vi "Goo0FF.vi"(10 "ColorSensor":dbl[](array[numeric])=[2.7490231560000002, 2.873534862, 2.8564450200000002, 2.873534862], 11 "클러스터":T1={{"정지할 차이값"=0.08, "흰색과 밖 차이값"=0.15, "흰/검 반 값 "=0.3}, {"4: 오른각도"=122.0, "4: 뒷쪽각도"=0.0, "5: 오른각도"=120.0, "5: 앞쪽각도"=245.0, "6: 왼쪽각도"=245.0, "6: 앞쪽각도"=120.0}, {"2: 공각도"=233.0, "2: 굴릴각도"=60.0}}) -> ()   [LabVIEW 2014]
uses:
  <vilib>/myRIO/Instrument Drivers/Onboard IO/AI/vis/Read.vi
  <vilib>/myRIO/Instrument Drivers/Onboard IO/AI/vis/Smart Open.vi
  <vilib>/Utility/error.llb/Error Cluster From Error Code.vi
  <vilib>/myRIO/Common/Instrument Driver Framework/myRIO v1.0/AI/vis/myRIO v1.0 Read AI.vi
panel:
  in  "오른쪽맞추는 초":u32=7000
  in  "오른쪽으로":u32=1000
  in  "왼쪽차이":dbl=0.25
  in  "Servo Position2 (0 - 255)":u8(slide)=115 step=1 scale=0.0..255.0
  in  "왼쪽가는 시간":u32=250
  in  "뒤로가는 시간":u32=100
  in  "Select Servo 2":string(combo)="Servo 2"
  in  "1: 정지":u8=128
  in  "1: 내리기":u8=10
  in  "1: 내리는 시간":u32=4000
  in  "Select Servo":string(combo)="Servo 1"
  in  "Select Servo 6":string(combo)="Servo 6"
  in  "Select Servo 5":string(combo)="Servo 5"
  in  "Select Servo 4":string(combo)="Servo 4"
  in  "서브 컨트롤":u8=1
  out "흰색과 밖 차이값":dbl=0.15
  # "마지막! 되돌아가기"
  # "115\n2번서브모터 본래방향"
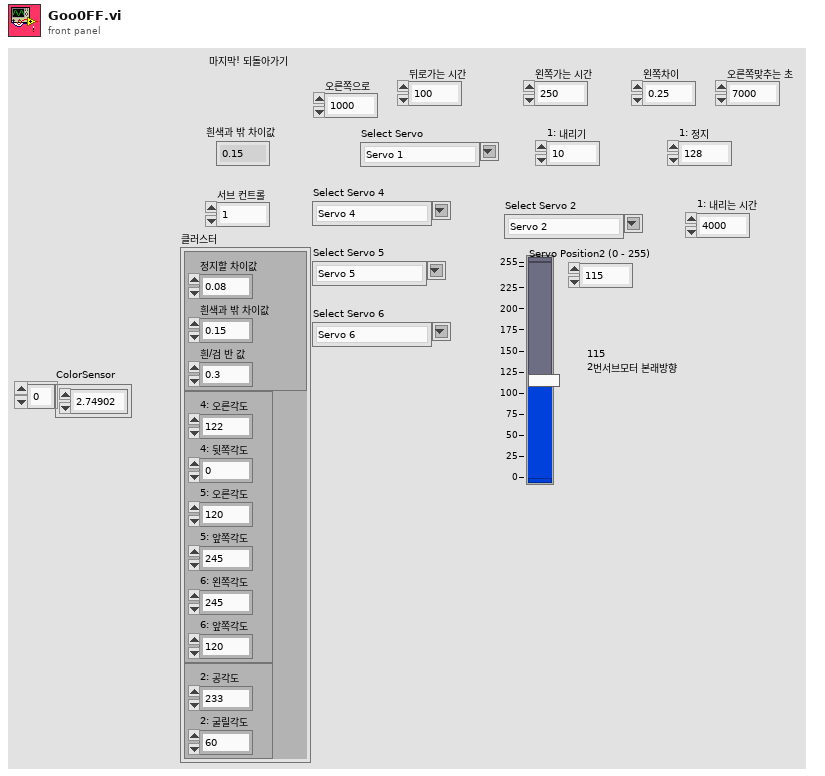
[diagram p1: front panel]
types:
  T1 = cluster{cluster{"정지할 차이값":dbl, "흰색과 밖 차이값":dbl, "흰/검 반 값 ":dbl}, cluster{"4: 오른각도":dbl, "4: 뒷쪽각도":dbl, "5: 오른각도":dbl, "5: 앞쪽각도":dbl, "6: 왼쪽각도":dbl, "6: 앞쪽각도":dbl}, cluster{"2: 공각도":dbl, "2: 굴릴각도":dbl}}
  T2 = cluster{"4: 오른각도":dbl, "4: 뒷쪽각도":dbl, "5: 오른각도":dbl, "5: 앞쪽각도":dbl, "6: 왼쪽각도":dbl, "6: 앞쪽각도":dbl}
  T3 = cluster{"정지할 차이값":dbl, "흰색과 밖 차이값":dbl, "흰/검 반 값 ":dbl}
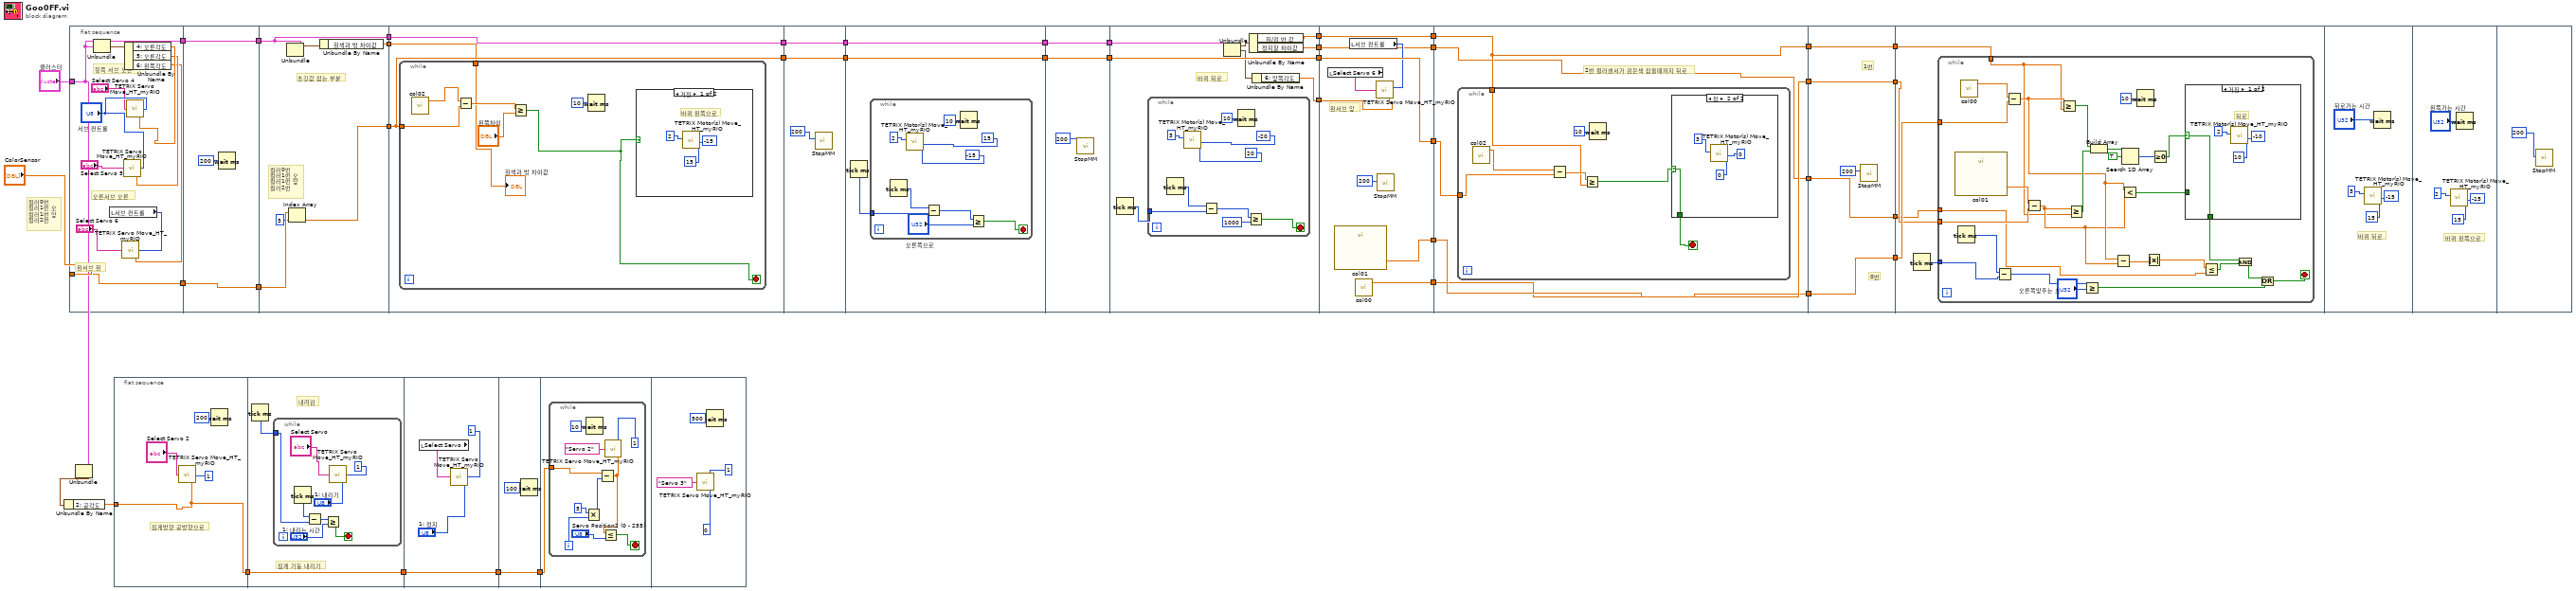
[diagram p0: block diagram]
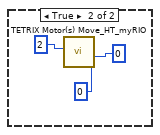
[diagram p2: hidden frame]
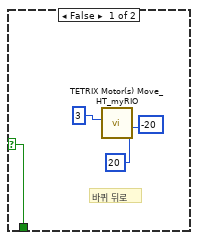
[diagram p3: hidden frame]
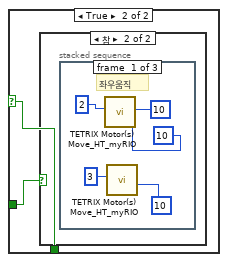
[diagram p4: hidden frame]
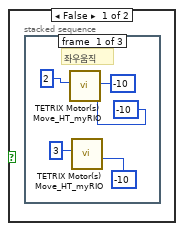
[diagram p5: hidden frame]
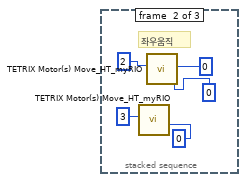
[diagram p6: hidden frame]
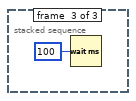
[diagram p7: hidden frame]
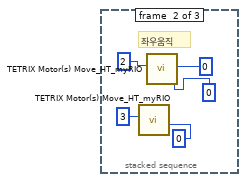
[diagram p8: hidden frame]
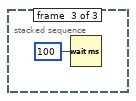
[diagram p9: hidden frame]
diagram:
  # "컬러0번\n컬러1번 오\n컬러1번 앞\n컬러2번"
  n1 = flat-sequence {
    tunnel: [w41] -> _
    tunnel: "클러스터" -> [w41]
    tunnel: [w42] -> w26
    tunnel: "ColorSensor" -> [w42]
    tunnel: [w41] -> w23
    tunnel: [w53] -> w27
    tunnel: w26 -> [w53]
    tunnel: [w52] -> w24
    tunnel: w23 -> [w52]
    tunnel: [w58] -> w40
    tunnel: w27 -> [w60]
    tunnel: w24 -> [w55]
    tunnel: [w56] -> w22
    tunnel: [w55] -> w21
    tunnel: w40 -> [w63]
    tunnel: [w63] -> w37
    tunnel: w22 -> [w62]
    tunnel: w21 -> [w61]
    tunnel: [w61] -> w20
    tunnel: w37 -> [w79]
    tunnel: [w79] -> w35
    tunnel: w20 -> [w77]
    tunnel: [w77] -> w19
    tunnel: w35 -> [w82]
    tunnel: [w82] -> w34
    tunnel: w19 -> [w81]
    tunnel: [w81] -> w18
    tunnel: w34 -> [w94]
    tunnel: [w94] -> w33
    tunnel: w18 -> [w92]
    tunnel: [w92] -> w17
    tunnel: w33 -> [w101]
    tunnel: [w101] -> w38
    tunnel: w17 -> [w100]
    tunnel: [w99] -> w16
    tunnel: [w96] -> w14
    tunnel: [w95] -> w3
    tunnel: [w120] -> w39
    tunnel: w38 -> [w120]
    tunnel: [w119] -> w36
    tunnel: [w118] -> w32
    tunnel: w16 -> [w114]
    tunnel: [w113] -> w15
    tunnel: w14 -> [w113]
    tunnel: [w112] -> w4
    tunnel: w3 -> [w112]
    tunnel: w39 -> [w125]
    tunnel: w36 -> [w124]
    tunnel: w32 -> [w123]
    tunnel: [w124] -> w30
    tunnel: [w123] -> w28
    tunnel: w15 -> [w122]
    tunnel: [w122] -> w5
    tunnel: w4 -> [w121]
    tunnel: [w121] -> w2
    tunnel: [w145] -> w31
    tunnel: w30 -> [w145]
    tunnel: [w144] -> w29
    tunnel: w28 -> [w144]
    tunnel: [w142] -> w6
    tunnel: w5 -> [w142]
    tunnel: w2 -> [w141]
    tunnel: [w141] -> w1
    tunnel: w31 -> [w149]
    tunnel: w29 -> [w150]
    tunnel: w6 -> [w148]
    tunnel: w1 -> [w147]
    frame #0 {
      # "왼서브 왼"
      # "오른서브 오른"
      # "뒷쪽 서브 오른"
      n2 = Unbundle(w41) -> (w46:T2)  [unwired: 2 out]
      n3 = local read "서브 컨트롤"() -> (w51:u8)
      n4 = Unbundle By Name(w46) -> ("4: 오른각도"=w45:dbl, "5: 오른각도"=w44:dbl, "6: 왼쪽각도"=w43:dbl)
      n5 = call <vilib>:"TETRIX Servo Move_HT_myRIO.vi"("Servo Position (0 - 255)"=w43, "Controller Daisy Chain Position (1 - 4)"=w51, "Select Servo"="Select Servo 6") -> ()  [unwired: 2 in, 1 out]
      n6 = call <vilib>:"TETRIX Servo Move_HT_myRIO.vi"("Servo Position (0 - 255)"=w44, "Controller Daisy Chain Position (1 - 4)"="서브 컨트롤", "Select Servo"="Select Servo 5") -> ()  [unwired: 2 in, 1 out]
      n7 = call <vilib>:"TETRIX Servo Move_HT_myRIO.vi"("Servo Position (0 - 255)"=w45, "Controller Daisy Chain Position (1 - 4)"="서브 컨트롤", "Select Servo"="Select Servo 4") -> ()  [unwired: 2 in, 1 out]
    }
    frame #1 {
      n8 = Wait (ms)(milliseconds to wait=u32 200 ("대기 시간(ms)")) -> ()  [unwired: 1 out]
    }
    frame #2 {
      # "컬러0번\n컬러1번 오\n컬러1번 앞\n컬러2번"
      # "초깃값 잡는 부분"
      n9 = Unbundle(w55) -> (w57:T3)  [unwired: 2 out]
      n10 = Index Array(array=w60, index=3 ("인덱스")) -> (element=w58:dbl)
      n11 = Unbundle By Name(w57) -> ("흰색과 밖 차이값"=w56:dbl)
    }
    frame #3 {
      n12 = while {
        tunnel: w63 -> [w70]
        tunnel: w62 -> [w64]
        stop <- w66 stop-if-true
        n13 = call "col02.vi"() -> ("Col02 (B/AI2 (Pin 7))"=w67:dbl)  [unwired: 26 in, 1 out]
        n14 = Subtract(x=w67, y=w70) -> (x-y=w69:dbl)
        n15 = Greater Or Equal?(x=w69, y="왼쪽차이") -> (x >= y?=w66:bool)
        n16 = Wait (ms)(milliseconds to wait=u32 10 ("대기 시간(ms)")) -> ()  [unwired: 1 out]
        n17 = case shown="거짓" w66 {
          frame False {
            # "바퀴 왼쪽으로"
            n18 = call <vilib>:"TETRIX Motor(s) Move_HT_myRIO.vi"("Motor 2 Power (-100 to 100)\n0 = Stop/Brake\n-128 = Stop/Coast"=i8 15 ("Motor 2 Power (-100 to 100)\n0 = Stop/Brake\n-128 = Stop/Coast"), "Motor 1 Power (-100 to 100)\n0 = Stop/Brake\n-128 = Stop/Coast"=i8 -15 ("Motor 1 Power (-100 to 100)\n0 = Stop/Brake\n-128 = Stop/Coast"), "Controller Daisy Chain Position: 1 - 4"=u8 2) -> ()  [unwired: 6 in, 1 out]
          }
          frame True {
            n19 = call <vilib>:"TETRIX Motor(s) Move_HT_myRIO.vi"("Motor 2 Power (-100 to 100)\n0 = Stop/Brake\n-128 = Stop/Coast"=i8 0 ("Motor 2 Power (-100 to 100)\n0 = Stop/Brake\n-128 = Stop/Coast"), "Motor 1 Power (-100 to 100)\n0 = Stop/Brake\n-128 = Stop/Coast"=i8 0 ("Motor 1 Power (-100 to 100)\n0 = Stop/Brake\n-128 = Stop/Coast"), "Controller Daisy Chain Position: 1 - 4"=u8 2) -> ()  [unwired: 6 in, 1 out]
          }
        }
        "흰색과 밖 차이값" <- w64
      }
    }
    frame #4 {
      n20 = call "StopMM.vi"("대기 시간(ms)"=u32 200) -> ()  [unwired: 11 in]
    }
    frame #5 {
      n21 = Tick Count (ms)() -> (millisecond timer value=w80:u32)
      n22 = while {
        tunnel: w80 -> [w87]
        stop <- w85 stop-if-true
        n23 = Tick Count (ms)() -> (millisecond timer value=w88:u32)
        n24 = call <vilib>:"TETRIX Motor(s) Move_HT_myRIO.vi"("Motor 2 Power (-100 to 100)\n0 = Stop/Brake\n-128 = Stop/Coast"=i8 -15 ("Motor 2 Power (-100 to 100)\n0 = Stop/Brake\n-128 = Stop/Coast"), "Motor 1 Power (-100 to 100)\n0 = Stop/Brake\n-128 = Stop/Coast"=i8 15 ("Motor 1 Power (-100 to 100)\n0 = Stop/Brake\n-128 = Stop/Coast"), "Controller Daisy Chain Position: 1 - 4"=u8 2) -> ()  [unwired: 6 in, 1 out]
        n25 = Subtract(x=w88, y=w87) -> (x-y=w86:u32)
        n26 = Wait (ms)(milliseconds to wait=u32 10 ("대기 시간(ms)")) -> ()  [unwired: 1 out]
        n27 = Greater Or Equal?(x=w86, y="오른쪽으로") -> (x >= y?=w85:bool)
      }
    }
    frame #6 {
      n28 = call "StopMM.vi"("대기 시간(ms)"=u32 200) -> ()  [unwired: 11 in]
    }
    frame #7 {
      # "바퀴 뒤로"
      n29 = Tick Count (ms)() -> (millisecond timer value=w102:u32)
      n30 = while {
        tunnel: w102 -> [w107]
        stop <- w104 stop-if-true
        n31 = Tick Count (ms)() -> (millisecond timer value=w108:u32)
        n32 = call <vilib>:"TETRIX Motor(s) Move_HT_myRIO.vi"("Motor 2 Power (-100 to 100)\n0 = Stop/Brake\n-128 = Stop/Coast"=i8 20 ("Motor 2 Power (-100 to 100)\n0 = Stop/Brake\n-128 = Stop/Coast"), "Motor 1 Power (-100 to 100)\n0 = Stop/Brake\n-128 = Stop/Coast"=i8 -20 ("Motor 1 Power (-100 to 100)\n0 = Stop/Brake\n-128 = Stop/Coast"), "Controller Daisy Chain Position: 1 - 4"=u8 3) -> ()  [unwired: 6 in, 1 out]
        n33 = Subtract(x=w108, y=w107) -> (x-y=w106:u32)
        n34 = Wait (ms)(milliseconds to wait=u32 10 ("대기 시간(ms)")) -> ()  [unwired: 1 out]
        n35 = Greater Or Equal?(x=w106, y=u32 1000) -> (x >= y?=w104:bool)
      }
      n36 = Unbundle(w100) -> (w97:T3, w98:T2)  [unwired: 1 out]
      n37 = Unbundle By Name(w97) -> ("흰/검 반 값"=w96:dbl, "정지할 차이값"=w95:dbl)
      n38 = Unbundle By Name(w98) -> ("6: 앞쪽각도"=w99:dbl)
    }
    frame #8 {
      # "왼서브 앞"
      n39 = local read "Select Servo 6"() -> (w116:string)
      n40 = call "col01.vi"() -> ("Col01 (B/AI1 (Pin 5))"=w119:dbl)  [unwired: 26 in, 1 out]
      n41 = local read "서브 컨트롤"() -> (w117:u8)
      n42 = call "col00.vi"() -> ("Col00 (B/AI0 (Pin 3))"=w118:dbl)  [unwired: 26 in, 1 out]
      n43 = call <vilib>:"TETRIX Servo Move_HT_myRIO.vi"("Servo Position (0 - 255)"=w114, "Controller Daisy Chain Position (1 - 4)"=w117, "Select Servo"=w116) -> ()  [unwired: 2 in, 1 out]
      n44 = call "StopMM.vi"("대기 시간(ms)"=u32 200) -> ()  [unwired: 11 in]
    }
    frame #9 {
      # "2번 컬러센서가 검은색 잡을때까지 뒤로"
      n45 = while {
        tunnel: w125 -> [w131]
        tunnel: w122 -> [w127]
        stop <- w126 stop-if-true
        n46 = call "col02.vi"() -> ("Col02 (B/AI2 (Pin 7))"=w130:dbl)  [unwired: 26 in, 1 out]
        n47 = Subtract(x=w130, y=w131) -> (x-y=w129:dbl)
        n48 = Greater Or Equal?(x=w129, y=w127) -> (x >= y?=w128:bool)
        n49 = Wait (ms)(milliseconds to wait=u32 10 ("대기 시간(ms)")) -> ()  [unwired: 1 out]
        n50 = case shown="참" w128 {
          selector: w128 -> [w133 w137]
          tunnel: [w133 w137] -> w126
          frame False {
            # "바퀴 뒤로"
            n51 = call <vilib>:"TETRIX Motor(s) Move_HT_myRIO.vi"("Motor 2 Power (-100 to 100)\n0 = Stop/Brake\n-128 = Stop/Coast"=i8 20 ("Motor 2 Power (-100 to 100)\n0 = Stop/Brake\n-128 = Stop/Coast"), "Motor 1 Power (-100 to 100)\n0 = Stop/Brake\n-128 = Stop/Coast"=i8 -20 ("Motor 1 Power (-100 to 100)\n0 = Stop/Brake\n-128 = Stop/Coast"), "Controller Daisy Chain Position: 1 - 4"=u8 3) -> ()  [unwired: 6 in, 1 out]
          }
          frame True {
            n52 = call <vilib>:"TETRIX Motor(s) Move_HT_myRIO.vi"("Motor 2 Power (-100 to 100)\n0 = Stop/Brake\n-128 = Stop/Coast"=i8 0 ("Motor 2 Power (-100 to 100)\n0 = Stop/Brake\n-128 = Stop/Coast"), "Motor 1 Power (-100 to 100)\n0 = Stop/Brake\n-128 = Stop/Coast"=i8 0 ("Motor 1 Power (-100 to 100)\n0 = Stop/Brake\n-128 = Stop/Coast"), "Controller Daisy Chain Position: 1 - 4"=u8 3) -> ()  [unwired: 6 in, 1 out]
          }
        }
      }
    }
    frame #10 {
      # "0번"
      # "1번"
      n53 = call "StopMM.vi"("대기 시간(ms)"=u32 200) -> ()  [unwired: 11 in]
    }
    frame #11 {
      n54 = Tick Count (ms)() -> (millisecond timer value=w146:u32)
      n55 = while {
        tunnel: w149 -> [w176]
        tunnel: w150 -> [w174]
        tunnel: w148 -> [w160]
        tunnel: w147 -> [w159]
        tunnel: w146 -> [w156]
        stop <- w153 stop-if-true
        n56 = call "col01.vi"() -> ("Col01 (B/AI1 (Pin 5))"=w177:dbl)  [unwired: 26 in, 1 out]
        n57 = Tick Count (ms)() -> (millisecond timer value=w157:u32)
        n58 = call "col00.vi"() -> ("Col00 (B/AI0 (Pin 3))"=w175:dbl)  [unwired: 26 in, 1 out]
        n59 = Subtract(x=w157, y=w156) -> (x-y=w155:u32)
        n60 = Subtract(x=w175, y=w174) -> (x-y=w163:dbl)
        n61 = Subtract(x=w177, y=w176) -> (x-y=w162:dbl)
        n62 = Greater Or Equal?(x=w163, y=w160) -> (x >= y?=w173:bool)
        n63 = Greater Or Equal?(x=w162, y=w160) -> (x >= y?=w172:bool)
        n64 = Greater Or Equal?(x=w155, y="오른쪽맞추는 초") -> (x >= y?=w152:bool)
        n65 = Build Array(w173, w172) -> (w171:bool[])
        n66 = Subtract(x=w163, y=w162) -> (x-y=w166:dbl)
        n67 = Search 1D Array(1D array=w171, element=TRUE ("원소")) -> (index of element=w169:i32)  [unwired: 1 in]
        n68 = Less?(x=w163, y=w162) -> (x < y?=w161:bool)
        n69 = Wait (ms)(milliseconds to wait=u32 10 ("대기 시간(ms)")) -> ()  [unwired: 1 out]
        n70 = Absolute Value(x=w166) -> (abs(x)=w165:dbl)
        n71 = Greater Or Equal To 0?(x=w169) -> (x >= 0?=w164:bool)
        n72 = case shown="거짓" w164 {
          selector: w164 -> [w178 w182]
          tunnel: w161 -> [_ w183]
          tunnel: [w178 w182] -> w158
          frame False {
            # "뒤로"
            n73 = call <vilib>:"TETRIX Motor(s) Move_HT_myRIO.vi"("Motor 2 Power (-100 to 100)\n0 = Stop/Brake\n-128 = Stop/Coast"=i8 10 ("Motor 2 Power (-100 to 100)\n0 = Stop/Brake\n-128 = Stop/Coast"), "Motor 1 Power (-100 to 100)\n0 = Stop/Brake\n-128 = Stop/Coast"=i8 -10 ("Motor 1 Power (-100 to 100)\n0 = Stop/Brake\n-128 = Stop/Coast"), "Controller Daisy Chain Position: 1 - 4"=u8 2) -> ()  [unwired: 6 in, 1 out]
          }
          frame True {
            n74 = case shown="참" w183 {
              frame False {
                n75 = stacked-sequence {
                  frame #0 {
                    # "좌우움직"
                    n76 = call <vilib>:"TETRIX Motor(s) Move_HT_myRIO.vi"("Motor 2 Power (-100 to 100)\n0 = Stop/Brake\n-128 = Stop/Coast"=i8 -10 ("Motor 2 Power (-100 to 100)\n0 = Stop/Brake\n-128 = Stop/Coast"), "Motor 1 Power (-100 to 100)\n0 = Stop/Brake\n-128 = Stop/Coast"=i8 -10 ("Motor 1 Power (-100 to 100)\n0 = Stop/Brake\n-128 = Stop/Coast"), "Controller Daisy Chain Position: 1 - 4"=u8 2) -> ()  [unwired: 6 in, 1 out]
                    n77 = call <vilib>:"TETRIX Motor(s) Move_HT_myRIO.vi"("Motor 1 Power (-100 to 100)\n0 = Stop/Brake\n-128 = Stop/Coast"=i8 -10 ("Motor 1 Power (-100 to 100)\n0 = Stop/Brake\n-128 = Stop/Coast"), "Controller Daisy Chain Position: 1 - 4"=u8 3) -> ()  [unwired: 7 in, 1 out]
                  }
                  frame #1 {
                    # "좌우움직"
                    n78 = call <vilib>:"TETRIX Motor(s) Move_HT_myRIO.vi"("Motor 1 Power (-100 to 100)\n0 = Stop/Brake\n-128 = Stop/Coast"=i8 0 ("Motor 1 Power (-100 to 100)\n0 = Stop/Brake\n-128 = Stop/Coast"), "Controller Daisy Chain Position: 1 - 4"=u8 3) -> ()  [unwired: 7 in, 1 out]
                    n79 = call <vilib>:"TETRIX Motor(s) Move_HT_myRIO.vi"("Motor 2 Power (-100 to 100)\n0 = Stop/Brake\n-128 = Stop/Coast"=i8 0 ("Motor 2 Power (-100 to 100)\n0 = Stop/Brake\n-128 = Stop/Coast"), "Motor 1 Power (-100 to 100)\n0 = Stop/Brake\n-128 = Stop/Coast"=i8 0 ("Motor 1 Power (-100 to 100)\n0 = Stop/Brake\n-128 = Stop/Coast"), "Controller Daisy Chain Position: 1 - 4"=u8 2) -> ()  [unwired: 6 in, 1 out]
                  }
                  frame #2 {
                    n80 = Wait (ms)(milliseconds to wait=u32 100 ("대기 시간(ms)")) -> ()  [unwired: 1 out]
                  }
                }
              }
              frame True {
                n81 = stacked-sequence {
                  frame #0 {
                    # "좌우움직"
                    n82 = call <vilib>:"TETRIX Motor(s) Move_HT_myRIO.vi"("Motor 2 Power (-100 to 100)\n0 = Stop/Brake\n-128 = Stop/Coast"=i8 10 ("Motor 2 Power (-100 to 100)\n0 = Stop/Brake\n-128 = Stop/Coast"), "Motor 1 Power (-100 to 100)\n0 = Stop/Brake\n-128 = Stop/Coast"=i8 10 ("Motor 1 Power (-100 to 100)\n0 = Stop/Brake\n-128 = Stop/Coast"), "Controller Daisy Chain Position: 1 - 4"=u8 2) -> ()  [unwired: 6 in, 1 out]
                    n83 = call <vilib>:"TETRIX Motor(s) Move_HT_myRIO.vi"("Motor 1 Power (-100 to 100)\n0 = Stop/Brake\n-128 = Stop/Coast"=i8 10 ("Motor 1 Power (-100 to 100)\n0 = Stop/Brake\n-128 = Stop/Coast"), "Controller Daisy Chain Position: 1 - 4"=u8 3) -> ()  [unwired: 7 in, 1 out]
                  }
                  frame #1 {
                    # "좌우움직"
                    n84 = call <vilib>:"TETRIX Motor(s) Move_HT_myRIO.vi"("Motor 1 Power (-100 to 100)\n0 = Stop/Brake\n-128 = Stop/Coast"=i8 0 ("Motor 1 Power (-100 to 100)\n0 = Stop/Brake\n-128 = Stop/Coast"), "Controller Daisy Chain Position: 1 - 4"=u8 3) -> ()  [unwired: 7 in, 1 out]
                    n85 = call <vilib>:"TETRIX Motor(s) Move_HT_myRIO.vi"("Motor 2 Power (-100 to 100)\n0 = Stop/Brake\n-128 = Stop/Coast"=i8 0 ("Motor 2 Power (-100 to 100)\n0 = Stop/Brake\n-128 = Stop/Coast"), "Motor 1 Power (-100 to 100)\n0 = Stop/Brake\n-128 = Stop/Coast"=i8 0 ("Motor 1 Power (-100 to 100)\n0 = Stop/Brake\n-128 = Stop/Coast"), "Controller Daisy Chain Position: 1 - 4"=u8 2) -> ()  [unwired: 6 in, 1 out]
                  }
                  frame #2 {
                    n86 = Wait (ms)(milliseconds to wait=u32 100 ("대기 시간(ms)")) -> ()  [unwired: 1 out]
                  }
                }
              }
            }
          }
        }
        n87 = Less Or Equal?(x=w165, y=w159) -> (x <= y?=w167:bool)
        n88 = And(x=w158, y=w167) -> (x .and. y?=w154:bool)
        n89 = Or(x=w154, y=w152) -> (x .or. y?=w153:bool)
      }
    }
    frame #12 {
      # "바퀴 뒤로"
      n90 = call <vilib>:"TETRIX Motor(s) Move_HT_myRIO.vi"("Motor 2 Power (-100 to 100)\n0 = Stop/Brake\n-128 = Stop/Coast"=i8 15 ("Motor 2 Power (-100 to 100)\n0 = Stop/Brake\n-128 = Stop/Coast"), "Motor 1 Power (-100 to 100)\n0 = Stop/Brake\n-128 = Stop/Coast"=i8 -15 ("Motor 1 Power (-100 to 100)\n0 = Stop/Brake\n-128 = Stop/Coast"), "Controller Daisy Chain Position: 1 - 4"=u8 3) -> ()  [unwired: 6 in, 1 out]
      n91 = Wait (ms)(milliseconds to wait="뒤로가는 시간") -> ()  [unwired: 1 out]
    }
    frame #13 {
      # "바퀴 왼쪽으로"
      n92 = call <vilib>:"TETRIX Motor(s) Move_HT_myRIO.vi"("Motor 2 Power (-100 to 100)\n0 = Stop/Brake\n-128 = Stop/Coast"=i8 15 ("Motor 2 Power (-100 to 100)\n0 = Stop/Brake\n-128 = Stop/Coast"), "Motor 1 Power (-100 to 100)\n0 = Stop/Brake\n-128 = Stop/Coast"=i8 -15 ("Motor 1 Power (-100 to 100)\n0 = Stop/Brake\n-128 = Stop/Coast"), "Controller Daisy Chain Position: 1 - 4"=u8 2) -> ()  [unwired: 6 in, 1 out]
      n93 = Wait (ms)(milliseconds to wait="왼쪽가는 시간") -> ()  [unwired: 1 out]
    }
    frame #14 {
      n94 = call "StopMM.vi"("대기 시간(ms)"=u32 200) -> ()  [unwired: 11 in]
    }
  }
  n95 = Unbundle("클러스터") -> (w12:cluster{"2: 공각도":dbl, "2: 굴릴각도":dbl})  [unwired: 2 out]
  n96 = Unbundle By Name(w12) -> ("2: 공각도"=w11:dbl)
  n97 = flat-sequence {
    tunnel: w11 -> [w215]
    tunnel: [w215] -> w7
    tunnel: [w219] -> w8
    tunnel: w7 -> [w219]
    tunnel: [w229] -> w9
    tunnel: w8 -> [w229]
    tunnel: [w233] -> w10
    tunnel: w9 -> [w233]
    tunnel: w10 -> [w235]
    frame #0 {
      # "집게방향 공방향으로"
      n98 = call <vilib>:"TETRIX Servo Move_HT_myRIO.vi"("Servo Position (0 - 255)"=w215, "Controller Daisy Chain Position (1 - 4)"=u8 1, "Select Servo"="Select Servo 2") -> ()  [unwired: 2 in, 1 out]
      n99 = Wait (ms)(milliseconds to wait=u32 200 ("대기 시간(ms)")) -> ()  [unwired: 1 out]
    }
    frame #1 {
      # "집게 기둥 내리기"
      # "내려감"
      n100 = Tick Count (ms)() -> (millisecond timer value=w220:u32)
      n101 = while {
        tunnel: w220 -> [w227]
        stop <- w225 stop-if-true
        n102 = Tick Count (ms)() -> (millisecond timer value=w228:u32)
        n103 = Subtract(x=w228, y=w227) -> (x-y=w226:u32)
        n104 = Greater Or Equal?(x=w226, y="1: 내리는 시간") -> (x >= y?=w225:bool)
        n105 = call <vilib>:"TETRIX Servo Move_HT_myRIO.vi"("Servo Position (0 - 255)"="1: 내리기", "Controller Daisy Chain Position (1 - 4)"=u8 1, "Select Servo"="Select Servo") -> ()  [unwired: 2 in, 1 out]
      }
    }
    frame #2 {
      n106 = local read "Select Servo"() -> (w231:string)
      n107 = call <vilib>:"TETRIX Servo Move_HT_myRIO.vi"("Servo Position (0 - 255)"="1: 정지", "Controller Daisy Chain Position (1 - 4)"=u8 1, "Select Servo"=w231) -> ()  [unwired: 2 in, 1 out]
    }
    frame #3 {
      n108 = Wait (ms)(milliseconds to wait=u32 100 ("대기 시간(ms)")) -> ()  [unwired: 1 out]
    }
    frame #4 {
      n109 = while {
        tunnel: w235 -> [w236]
        i -> [w242]
        stop <- w241 stop-if-true
        n110 = Multiply(x=u8 5 ("Servo Position (0 - 255)"), y=w242) -> (x*y=w240:i32)
        n111 = Wait (ms)(milliseconds to wait=u32 10 ("대기 시간(ms)")) -> ()  [unwired: 1 out]
        n112 = Subtract(x=w236, y=w240) -> (x-y=w239:dbl)
        n113 = Less Or Equal?(x=w239, y="Servo Position2 (0 - 255)") -> (x <= y?=w241:bool)
        n114 = call <vilib>:"TETRIX Servo Move_HT_myRIO.vi"("Servo Position (0 - 255)"=w239, "Controller Daisy Chain Position (1 - 4)"=u8 1, "Select Servo"="Servo 2") -> ()  [unwired: 2 in, 1 out]
      }
    }
    frame #5 {
      n115 = call <vilib>:"TETRIX Servo Move_HT_myRIO.vi"("Servo Position (0 - 255)"=u8 0, "Controller Daisy Chain Position (1 - 4)"=u8 1, "Select Servo"="Servo 3") -> ()  [unwired: 2 in, 1 out]
      n116 = Wait (ms)(milliseconds to wait=u32 500 ("대기 시간(ms)")) -> ()  [unwired: 1 out]
    }
  }
